vi "FINAL.vi"() -> ()   [LabVIEW 2020]
panel:
  out "error out":errorcluster
  out "Original 2":T1(plugin-control) caption="Original Image"
  out "Área de particulas":T2(graph)
  out "ROJO":bool
  out "AMBAR":bool
  out "VERDE":bool
  out "Área de particualas total":dbl
  out "Number of Particles":i32
  in  "name or relative path":path=path "C:/Users/axel2/OneDrive/Documents/Ejercicios_Labview/Topicos Selectos/Proyecto/Ex3_ComSerial_Ard_LV/mexico_tmo_2013066_lrg.jpg"
  out "Particle Reports (Real-World)":T3(array[cluster]) {"Orientation" format="%.2f"; "Dimensions"."Height" format="%.2f"; "Dimensions"."Width" format="%.2f"; "Center of Mass"."Y" format="%.2f"; "Center of Mass"."X" format="%.2f"; "Bounding Rect"."Bottom" format="%.2f"; "Bounding Rect"."Right" format="%.2f"; "Bounding Rect"."Top" format="%.2f"; "Bounding Rect"."Left" format="%.2f"; "Number of Holes" format="%.2f"; "Area" format="%.2f"}
  out "Señales Analógicas":dynamicdata(graph)
  out "Señales Digitales":dynamicdata(graph)
  out "Cluster Señales":T4
  out "LISTO?":bool=TRUE
  out "Buffer Filtrado":string
  out "Buffer Completo":string
  in  "Decisión":bool
  in  "stop":bool
  in  "Comando":T5(ring)
  in  "error in (no error)":errorcluster
  in  "VISA resource name":refnum<visa-resource-name>
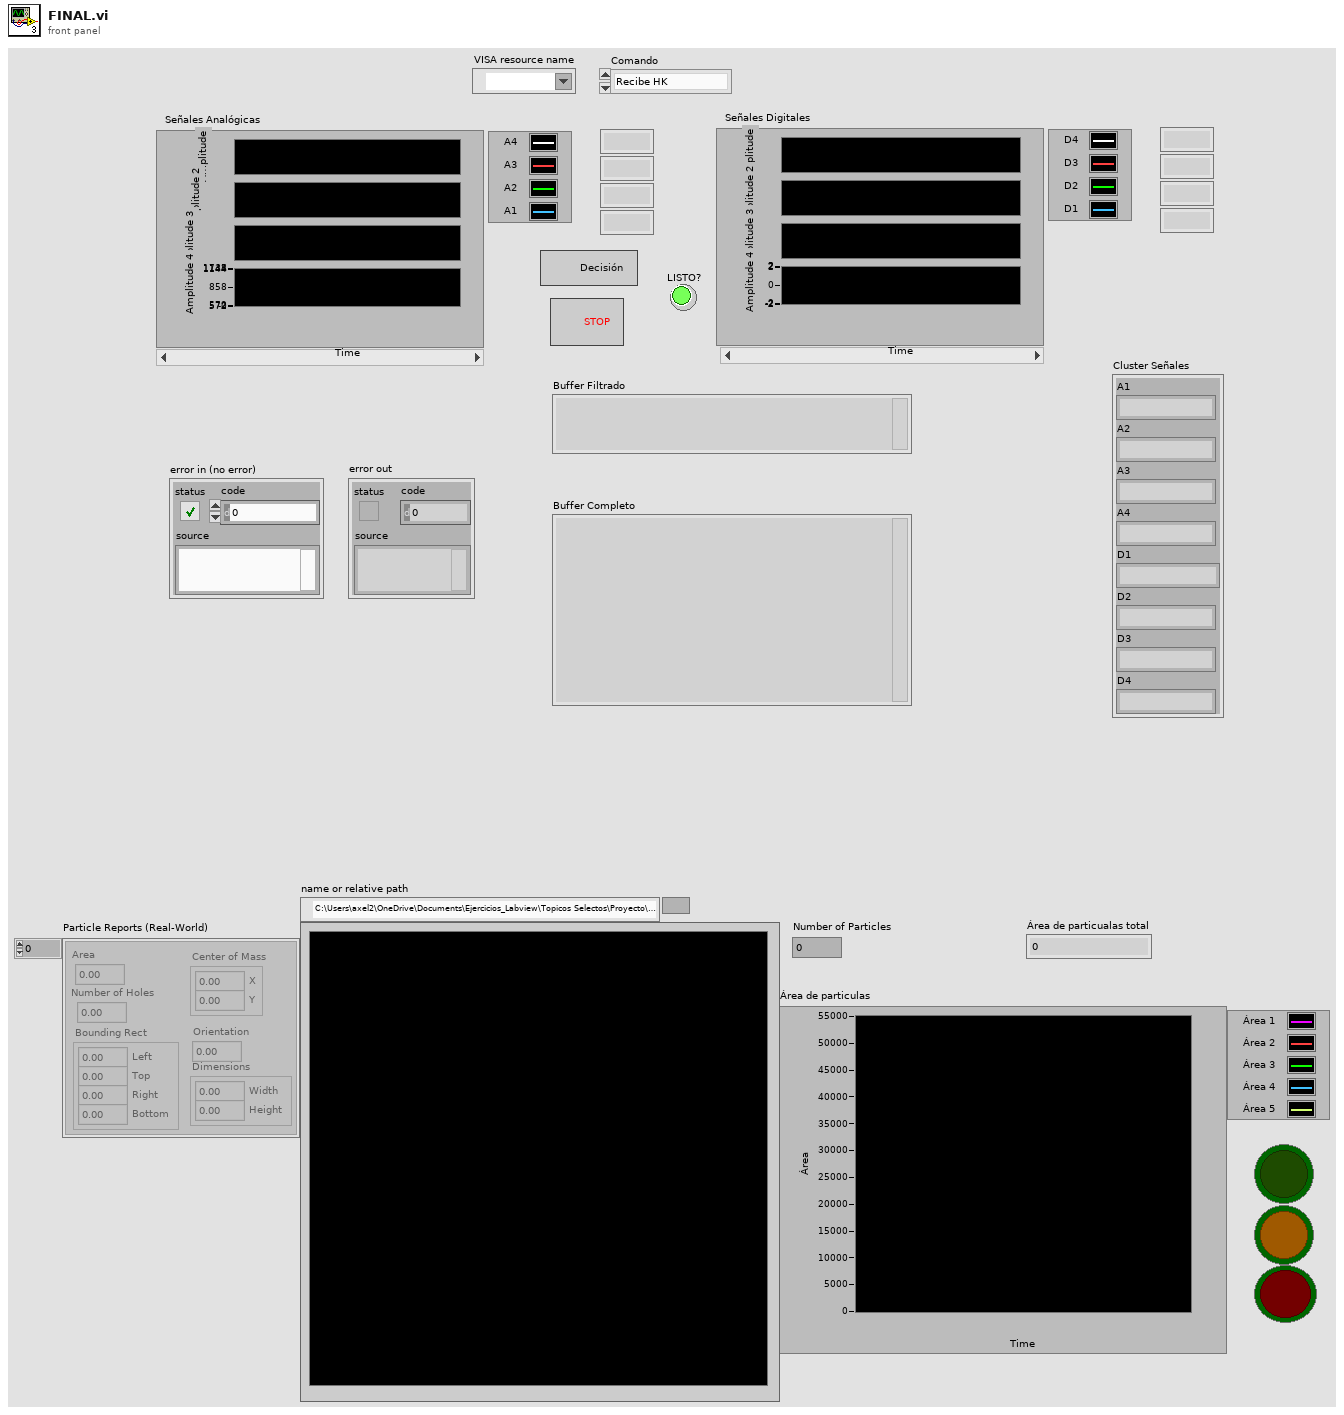
[diagram p1: front panel]
types:
  T1 = typedef "IMAQ Image.ctl" = refnum<image>
  T2 = cluster{"Area":dbl, "Area":dbl, "Area":dbl, "Area":dbl, "Area":dbl, "Area":dbl}
  T3 = cluster{"Area":dbl, "Number of Holes":dbl, "Bounding Rect":cluster{"Left":dbl, "Top":dbl, "Right":dbl, "Bottom":dbl}, "Center of Mass":cluster{"X":dbl, "Y":dbl}, "Orientation":dbl, "Dimensions":cluster{"Width":dbl, "Height":dbl}}[]
  T4 = cluster{"A1":string, "A2":string, "A3":string, "A4":string, "D1":string, "D2":string, "D3":string, "D4":string}
  T5 = enum16{"Recibe HK", "Act Fecha", "Parametros", "Reset", "Stop"}
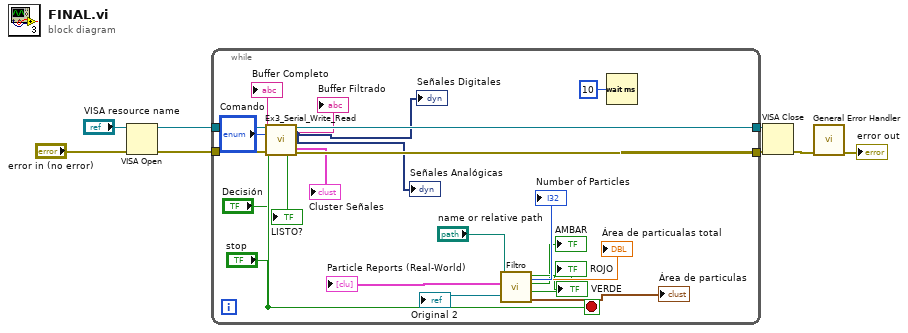
[diagram p0: block diagram]
diagram:
  n1 = VISA Open(error in (no error)="error in (no error)", VISA resource name="VISA resource name") -> (VISA resource name=w8:refnum<visa-resource-name>, error out=w5:errorcluster)  [unwired: 3 in]
  n2 = while {
    tunnel: w8 -> [w30]
    tunnel: w5 -> [w29]
    tunnel: [w28] -> w4
    tunnel: [w27] -> w3
    stop <- "stop" stop-if-true
    n3 = call "Ex3_Serial_Write_Read.vi"("VISA resource"=w30, "Comando"="Comando", "stop"="stop", "Decisión"="Decisión", "error in (no error)"=w29) -> ("Buffer Completo"=→"Buffer Completo":string, "Buffer Filtrado"=→"Buffer Filtrado":string, "VISA resource name out"=w27:refnum<visa-resource-name>, "Señales Digitales"=→"Señales Digitales" →"Señales Analógicas":dynamicdata, "LISTO?"=→"LISTO?":bool, "Cluster Señales"=→"Cluster Señales":T4, "error out"=w28:errorcluster)  [unwired: 3 in, 1 out]
    n4 = call "Filtro.vi"("name or relative path 2"="name or relative path") -> ("Área de particulas"=→"Área de particulas":T2, "ROJO"=→"ROJO":bool, "AMBAR"=→"AMBAR":bool, "VERDE"=→"VERDE":bool, "Original 2"=→"Original 2":T1, "Área de particualas total"=→"Área de particualas total":dbl, "Number of Particles 2"=→"Number of Particles":i32, "Particle Reports (Real-World)"=→"Particle Reports (Real-World)":T3)  [unwired: 3 in]
    n5 = Wait (ms)(milliseconds to wait=u32 10) -> ()  [unwired: 1 out]
  }
  n6 = VISA Close(VISA resource name=w3, error in (no error)=w4) -> (error out=w2:errorcluster)
  n7 = call <vilib>:"General Error Handler.vi"("error in (no error)"=w2) -> ("error out"=→"error out":errorcluster)  [unwired: 10 in, 4 out]
